vi "Subsystem.vi"(4 "L(m) in":dbl(slide) scale=0.0..10.0, 6 "M(kg) in":dbl(slide) scale=0.0..10.0, 7 "initial position in":dbl(slide) scale=-1.5..1.5, 9 "B(Nms/rad) in":dbl(slide) scale=0.0..50.0, 10 "Tau(Nm) in":dbl(slide) scale=-10.0..10.0, 11 "initial velocity in":dbl(slide) scale=-10.0..10.0) -> (0 "J 2":dbl, 1 "theta":dbl, 2 "dtheta":dbl, 3 "ddtheta":dbl, 5 "mlg/2 2":dbl)   [LabVIEW 2019]
uses:
  <vilib>/Simulation/Implementation/Shared/SIMSCR Execution Mode.ctl
  <vilib>/Simulation/Scripting/Companion Diagram/SimConfigNode/SimParams.ctl
  <vilib>/Simulation/Scripting/Companion Diagram/SimConfigNode/_simSolvers.ctl
  <vilib>/Simulation/Param Hierarchy/Typedefs/SIMPH Param Control Actions.ctl
  <vilib>/Simulation/Implementation/Shared/SIM limit type.ctl
  <vilib>/Simulation/Implementation/Shared/NILVSim_ParamChanged.vi
  <vilib>/Simulation/Implementation/Shared/NILVSIM_BeginStep.vi
  <vilib>/Simulation/ContinuousLinear/Implementation/NILVSim Integrator new.llb/SIM Integrator distributor (scalar).vi
  <vilib>/Simulation/SignalArithmetic/Implementation/NILVSim Gain.llb/SIM Gain (scalar).vi
  <vilib>/Simulation/ContinuousLinear/Implementation/NILVSim Integrator new.llb/SIM Integrator collector (scalar).vi
  <vilib>/Simulation/Implementation/Shared/NILVSim_Manager.vi
  <vilib>/Utility/error.llb/Clear Errors.vi
  <vilib>/Simulation/Implementation/Shared/NILVSim_FinalizeModel.vi
  <vilib>/Simulation/Implementation/Shared/SIM Unbundle Sim Info.vi
  <vilib>/Simulation/Implementation/Shared/SIMSH Read Queue.vi
  <vilib>/Simulation/Implementation/Shared/NILVSim_Initialize.vi
  <vilib>/Simulation/Utility/Implementation/NILVSim Get Time and IsAcceptedStep.vi
  <vilib>/Simulation/Implementation/Shared/NILVSim_GetModelError.vi
  <vilib>/Simulation/Implementation/Shared/SIM SimErrorHandler.vi
  <vilib>/Simulation/Implementation/Shared/SIM Bundle Sim Info.vi
  <vilib>/Simulation/Scripting/Companion Diagram/SimConfigNode/SimDog.xnode
  <vilib>/Simulation/Implementation/XNodeFramework/SimXNode/SimX.xnode
  <vilib>/Simulation/ContinuousLinear/Implementation/NILVSim Integrator new.llb/SIM Integrator (scalar).vi
  <vilib>/Simulation/Implementation/Shared/NI_SIM_Implementation.lvlib
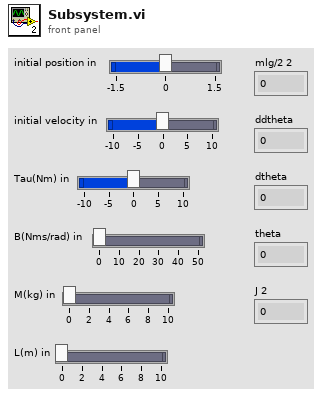
[diagram p1: front panel]
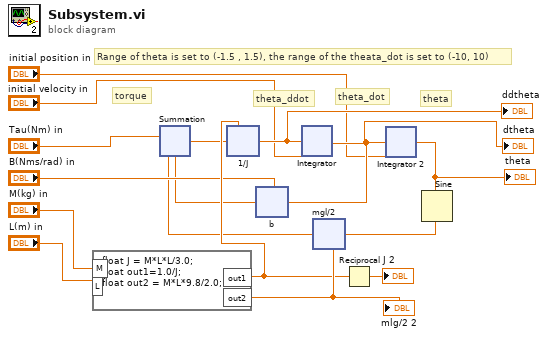
[diagram p0: block diagram]
diagram:
  # "Range of theta is set to (-1.5 , 1.5), the range of the theata_dot is set to (-10, 10)"
  # "theta"
  # "torque"
  # "theta_ddot"
  # "theta_dot"
  n1 = formula code="float J = M*L*L/3.0;\nfloat out1=1.0/J;\nfloat out2 = M*L*9.8/2.0;"("M"="M(kg) in", "L"="L(m) in") -> ("out1"=w9:dbl, "out2"=w13:dbl)
  "mlg/2 2" <- w13
  n2 = Reciprocal(x=w9) -> (1/x=→"J 2":dbl)
  n3 = xnode "Summation"("Operand1"="Tau(Nm) in", "Operand2"=w3, "Operand3"=w2) -> ("Result"=w6:dbl)
  n4 = xnode "1/J"("gain"=w9, "input"=w6) -> ("output"=w16:dbl)  [unwired: 2 in]
  "ddtheta" <- w16
  n5 = xnode "Integrator"("input"=w16, "initial condition"="initial velocity in") -> ("output"=w15:dbl)  [unwired: 8 in, 2 out]
  "dtheta" <- w15
  n6 = xnode "b"("gain"="B(Nms/rad) in", "input"=w15) -> ("output"=w2:dbl)  [unwired: 2 in]
  n7 = xnode "Integrator 2"("input"=w15, "initial condition"="initial position in") -> ("output"=w14:dbl)  [unwired: 8 in, 2 out]
  "theta" <- w14
  n8 = Sine(x=w14) -> (sin(x)=w4:dbl)
  n9 = xnode "mgl/2"("gain"=w13, "input"=w4) -> ("output"=w3:dbl)  [unwired: 2 in]
